vi "写入钻床基本操作.lvclass.vi"(8 "error in (no error)":errorcluster caption="错误输入（无错误）", 10 "钻床基本操作.lvclass":refnum<class "钻床基本操作.lvclass">, 11 "命令：打开冷却输入":refnum<class "命令：关闭冷却.lvclass">) -> (0 "error out":errorcluster caption="错误输出", 3 "命令：打开冷却输出":refnum<class "命令：关闭冷却.lvclass">)   [LabVIEW 2011, in "命令：关闭冷却.lvclass"]
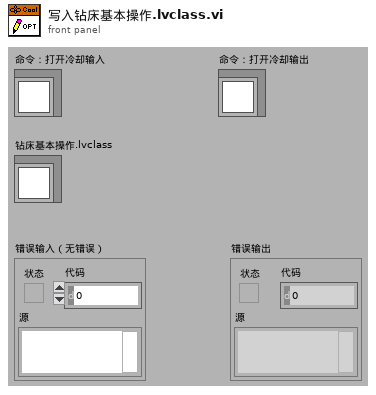
[diagram p1: front panel]
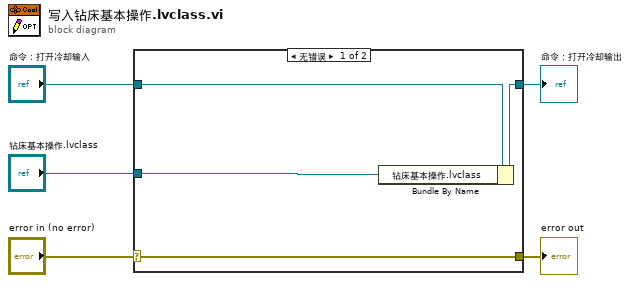
[diagram p0: block diagram]
diagram:
  n1 = case shown="无错误" "error in (no error)" {
    selector: "error in (no error)" -> [w9 w10]
    tunnel: [w9 w10] -> w4
    tunnel: [w7 w11] -> w2
    tunnel: "命令：打开冷却输入" -> [w8 w11]
    tunnel: "钻床基本操作.lvclass" -> [w6 _]
    frame No Error {
      n2 = Bundle By Name(cluster=w8, "钻床基本操作.lvclass"=w6) -> (w7:refnum<class "命令：关闭冷却.lvclass">)
    }
    frame Error {
    }
  }
  "error out" <- w4
  "命令：打开冷却输出" <- w2
